vi "Class - ResultCntr.SubSectionEnd.vi"(8 "error in (no error)":errorcluster, 11 "Class - ResultCntr in":refnum<class "Class - ResultCntr.lvclass">) -> (0 "error out":errorcluster, 1 "ID":string, 3 "Class - ResultCntr out":refnum<class "Class - ResultCntr.lvclass">)   [LabVIEW 2024, in "EQMF.lvlib" / "Results.lvlib" / "Class - ResultCntr.lvclass"]
uses:
  Class - ResultCntr.lvclass
  Class - ResultCntr.lvclass/Class - ResultCntr.ctl
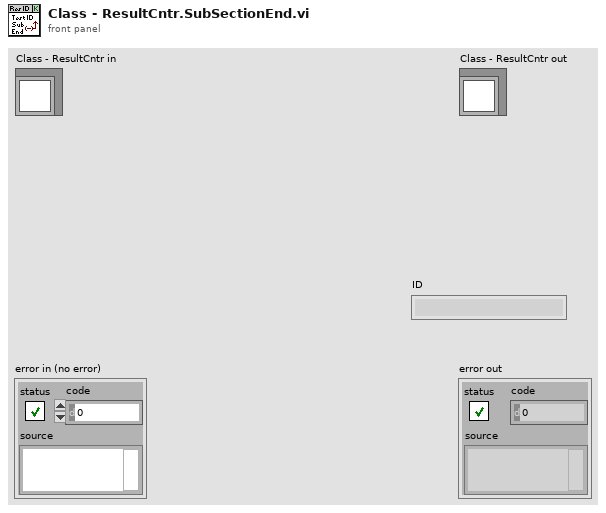
[diagram p1: front panel]
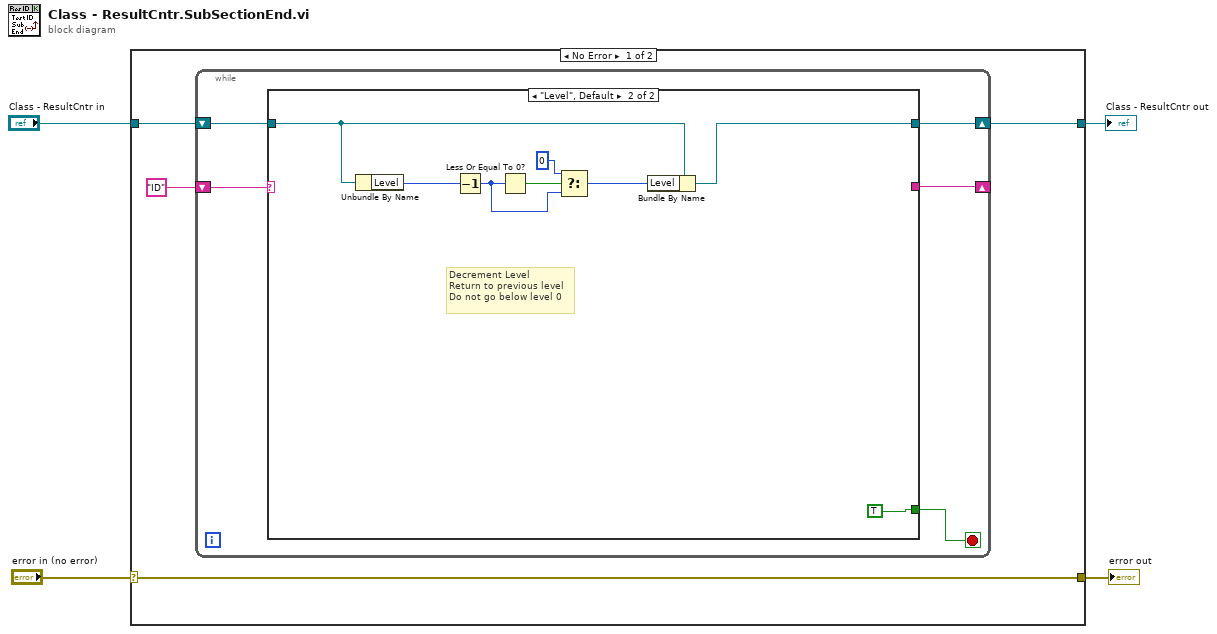
[diagram p0: block diagram]
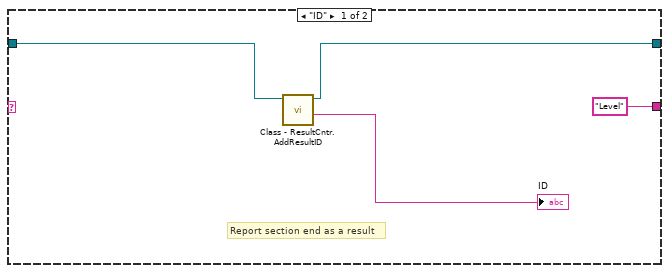
[diagram p2: hidden frame]
diagram:
  n1 = case shown="No Error" "error in (no error)" {
    selector: "error in (no error)" -> [w8 w27]
    tunnel: [w8 w27] -> w3
    tunnel: [w5 w26] -> w1
    tunnel: "Class - ResultCntr in" -> [w7 w26]
    frame No Error {
      n2 = while {
        shift-right: [w11] -> w5
        shift-left: w7 -> [w12]
        shift-right: [w10] -> _
        shift-left: "ID" -> [w13]
        stop <- w9 stop-if-true
        n3 = case shown="\"Level\", Default" w13 {
          tunnel: w12 -> [w17 w25]
          tunnel: [w16 w24] -> w11
          tunnel: ["Level" _] -> w10
          tunnel: [_ TRUE] -> w9
          frame "ID" {
            # "Report section end as a result"
            n4 = call "Class - ResultCntr.AddResultID.vi"("Class - ResultCntr in"=w17) -> ("ID"=→"ID":string, "Class - ResultCntr out"=w16:refnum<class "Class - ResultCntr.lvclass">)  [unwired: 8 in, 1 out]
          }
          frame "Level", Default {
            # "Decrement Level\nReturn to previous level\nDo not go below level 0"
            n5 = Unbundle By Name(w25) -> ("Level"=w19:i32)
            n6 = Decrement(x=w19) -> (x-1=w21:i32)
            n7 = Less Or Equal To 0?(x=w21) -> (x <= 0?=w23:bool)
            n8 = Select(t=0, s=w23, f=w21) -> (s? t:f=w22:i32)
            n9 = Bundle By Name(cluster=w25, "Level"=w22) -> (w24:refnum<class "Class - ResultCntr.lvclass">)
          }
        }
      }
    }
    frame Error {
    }
  }
  "error out" <- w3
  "Class - ResultCntr out" <- w1
